vi "关闭队列.vi"(8 "error in (no error)":errorcluster, 11 "输出簇":T1) -> (0 "error out":errorcluster)   [LabVIEW 2015]
uses:
  <vilib>/vision/Image Controls.llb/IMAQ Image.ctl
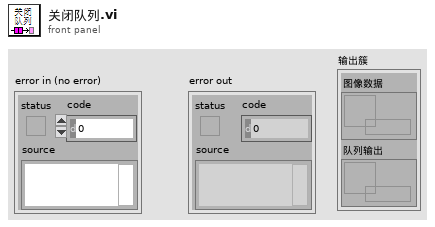
[diagram p1: front panel]
types:
  T1 = cluster{"图像数据":refnum<queue>, "队列输出":refnum<queue>}
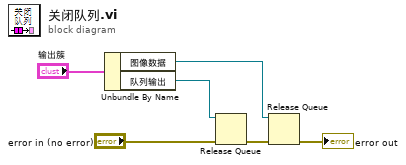
[diagram p0: block diagram]
diagram:
  n1 = Unbundle By Name("输出簇") -> ("图像数据"=w1:refnum<queue>, "队列输出"=w2:refnum<queue>)
  n2 = Release Queue(queue=w2, error in (no error)="error in (no error)") -> (error out=w3:errorcluster)  [unwired: 3 out]
  n3 = Release Queue(queue=w1, error in (no error)=w3) -> (error out=→"error out":errorcluster)  [unwired: 3 out]
